vi "Verify Account.vi"(8 "error in (no error)":errorcluster, 10 "Account Number":string, 11 "Account Database in":refnum<class "Account Database.lvclass">) -> (0 "error out":errorcluster, 1 "Account Data":T1, 2 "Valid Account Number?":bool, 3 "Account Database out":refnum<class "Account Database.lvclass">)   [LabVIEW 2020, in "Account Database.lvclass"]
uses:
  Account Database.lvclass
  Account Data.ctl
  Account Database.lvclass/Account Database.ctl
  <vilib>/Utility/file.llb/Read Delimited Spreadsheet (string).vi
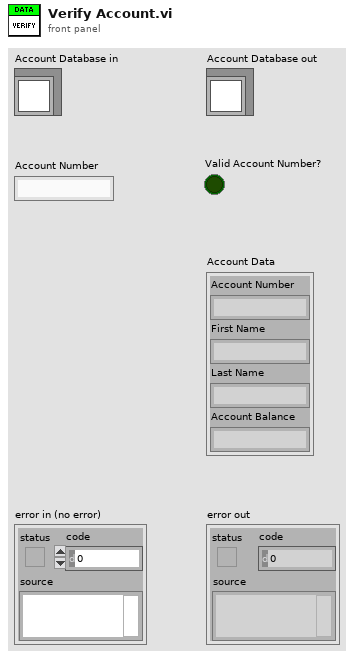
[diagram p1: front panel]
types:
  T1 = typedef "Account Database.lvclass/Account Data.ctl" = cluster{"Account Number":string, "First Name":string, "Last Name":string, "Account Balance":string}
  T2 = cluster{"all rows[0]":string, "all rows[1]":string, "all rows[2]":string, "all rows[3]":string}
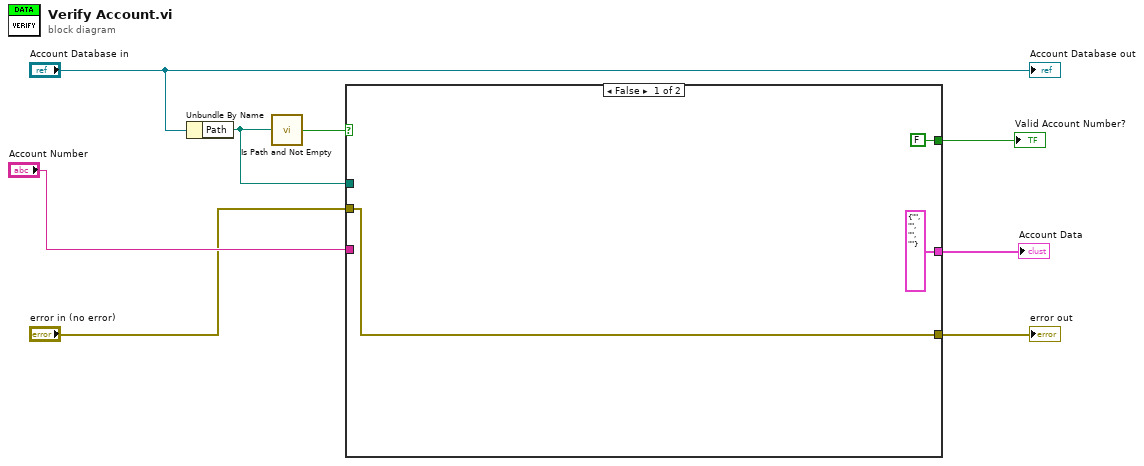
[diagram p0: block diagram]
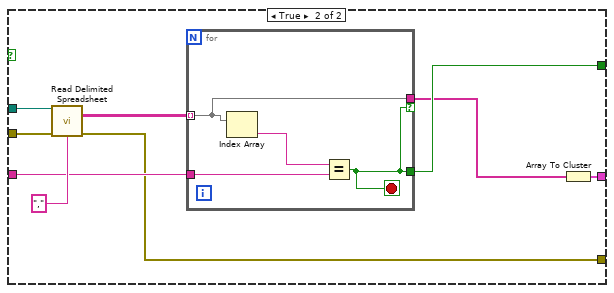
[diagram p2: hidden frame]
diagram:
  n1 = Unbundle By Name("Account Database in") -> ("Path"=w2:path)
  n2 = call <vilib>:"Is Path and Not Empty.vi"("path"=w2) -> ("Is Path and Not Empty?"=w1:bool)  [unwired: 4 in]
  n3 = case shown="False" w1 {
    tunnel: "Account Number" -> [_ w18]
    tunnel: [FALSE w17] -> w6
    tunnel: "error in (no error)" -> [w9 w16]
    tunnel: [w9 w15] -> w4
    tunnel: [T2 {"all rows[0]"="", "all rows[1]"="", "all rows[2]"="", "all rows[3]"=""} ("all rows") w13] -> w3
    tunnel: w2 -> [_ w12]
    frame False {
    }
    frame True {
      n4 = call-poly <vilib>:"Read Delimited Spreadsheet.vi"("file path (dialog if empty)"=w12, "error in (no error)"=w16, "delimiter (\\t)"="," ("delimiter (\\t)")) -> ("all rows"=w20:string[][], "error out"=w15:errorcluster)  [unwired: 7 in, 4 out]
      n5 = for {
        tunnel: w20 -> [w22] mode=indexing
        tunnel: w18 -> [w24]
        tunnel: [w21] -> w17
        tunnel: [w22] -> w14 if=w21
        stop <- w21 stop-if-true
        n6 = Index Array(array=w22) -> (element=w23:string)  [unwired: 1 in]
        n7 = Equal?(x=w23, y=w24) -> (x = y?=w21:bool)
      }
      n8 = Array To Cluster(array=w14) -> (cluster=w13:T2)
    }
  }
  "error out" <- w4
  "Valid Account Number?" <- w6
  "Account Data" <- w3
  "Account Database out" <- "Account Database in"
